vi "Boolean Trigger.vi"(0 "input":bool) -> (2 "rising edge":bool, 3 "falling edge":bool)   [LabVIEW 2011]
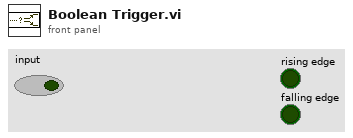
[diagram p1: front panel]
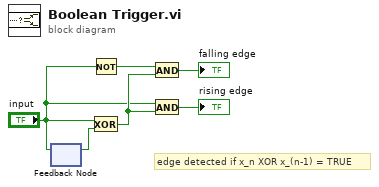
[diagram p0: block diagram]
diagram:
  # "edge detected if x_n XOR x_(n-1) = TRUE"
  n1 = feedback-in #1("input") -> ()
  n2 = feedback #1() -> (w6:bool)  [unwired: 1 in]
  n3 = Not(x="input") -> (.not. x?=w5:bool)
  n4 = Exclusive Or(1:w6, 2:"input") -> (0:w4:bool)
  n5 = And(x=w5, y=w4) -> (x .and. y?=→"falling edge":bool)
  n6 = And(x="input", y=w4) -> (x .and. y?=→"rising edge":bool)
